vi "Register Click Event Callback.vi"(8 "error in":errorcluster, 9 "onClick":refnum<user-event>, 10 "onClick Callback":refnum<vi>, 11 "Custom Events in":refnum<class "Custom Events.lvclass">) -> (0 "error out":errorcluster, 3 "Custom Events out":refnum<class "Custom Events.lvclass">)   [LabVIEW 2024, in "SourceGrid.lvlib" / "Custom Events.lvclass"]
uses:
  Custom Events.lvclass
  Custom Events.lvclass/Custom Events.ctl
  D:/git/Sourcegrid-LabVIEW/dll/SourceGrid.dll
  dll/SourceGrid.dll
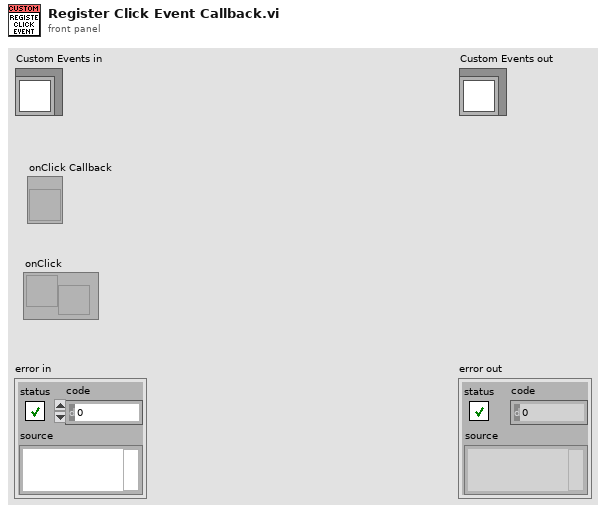
[diagram p1: front panel]
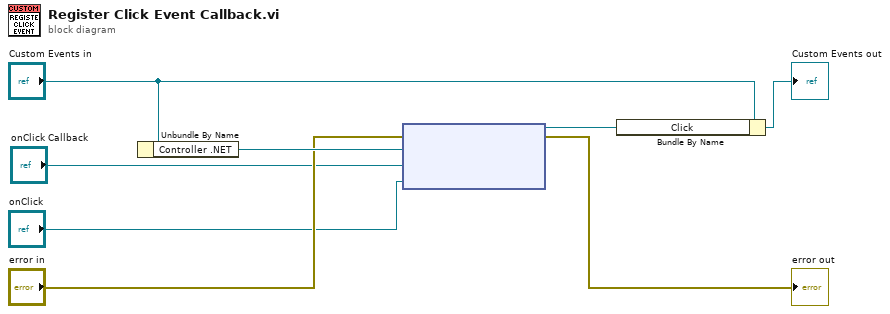
[diagram p0: block diagram]
diagram:
  n1 = Unbundle By Name("Custom Events in") -> ("Controller .NET"=w8:refnum<k24>)
  n2 = node("error in", w8, "onClick Callback", "onClick") -> (w3:refnum<k27>, →"error out":errorcluster)  [unwired: 1 in]
  n3 = Bundle By Name(cluster="Custom Events in", "Click"=w3) -> (→"Custom Events out":refnum<class "Custom Events.lvclass">)
